vi "ElmoDigIn2HomeFlag.vi"(1 "Digital Input (I32)":i32) -> (0 "Home Flag":bool)   [LabVIEW 2018]
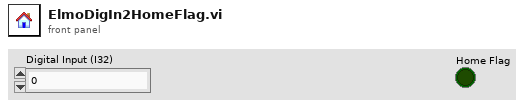
[diagram p1: front panel]
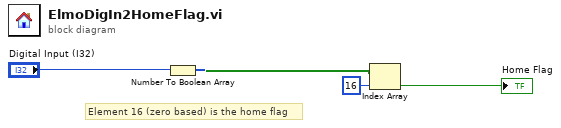
[diagram p0: block diagram]
diagram:
  # "Element 16 (zero based) is the home flag"
  n1 = Number To Boolean Array(number="Digital Input (I32)") -> (Boolean array=w3:bool[])
  n2 = Index Array(array=w3, index=16) -> (element=→"Home Flag":bool)
